vi "LumberjackConfigFromDTO.vi"(8 "error in (no error)":errorcluster, 11 "LumberjackConfigDTO":T9={"schemaVersion"="", "globalThreshold"="INFO", "defaultFileAppender"={"common"={"id"="", "threshold"="INFO", "filter"={"mode"="mirror", "levelMin"="INFO", "levelMax"="INFO", "tagPrefix"=""}, "queueBound"=0, "dropPolicy"="dropOldest", "useUTC"=FALSE}, "file"={"rootFolder"="", "maxFileSize"=0, "maxFileCount"=0, "baseName"="", "extension"="", "delimiter"="", "calendarFolderTree"=FALSE}}}) -> (0 "error out":errorcluster, 3 "LumberjackConfig":T1={"schemaVersion"="", "globalThreshold"=enum."INFO", "defaultFileAppender"={"common"={"id"="", "threshold"=enum."INFO", "filter"={"mode"=enum."Mirror", "levelMin"=enum."INFO", "levelMax"=enum."INFO", "tagPrefix"=""}, "queueBound"=0, "dropPolicy"=enum."DropOldest", "useUTC"=FALSE}, "file"={"rootFolder"=path "", "maxFileSize"=0, "maxFileCount"=0, "baseName"="", "extension"="", "delimiter"="", "calendarFolderTree"=FALSE}}})   [LabVIEW 2026, in "Lumberjack.lvlib"]
uses:
  Lumberjack.lvlib
  TypeDefs/Severity.ctl
  TypeDefs/FilterMode.ctl
  TypeDefs/Filter.ctl
  TypeDefs/DropPolicy.ctl
  TypeDefs/AppenderConfig.ctl
  TypeDefs/FileAppenderConfig.ctl
  TypeDefs/LumberjackConfig.ctl
  TypeDefs/FileConfig.ctl
  TypeDefs/ConfigDTO/FilterDTO.ctl
  TypeDefs/ConfigDTO/AppenderConfigDTO.ctl
  TypeDefs/ConfigDTO/FileAppenderConfigDTO.ctl
  TypeDefs/ConfigDTO/LumberjackConfigDTO.ctl
  TypeDefs/ConfigDTO/FileConfigDTO.ctl
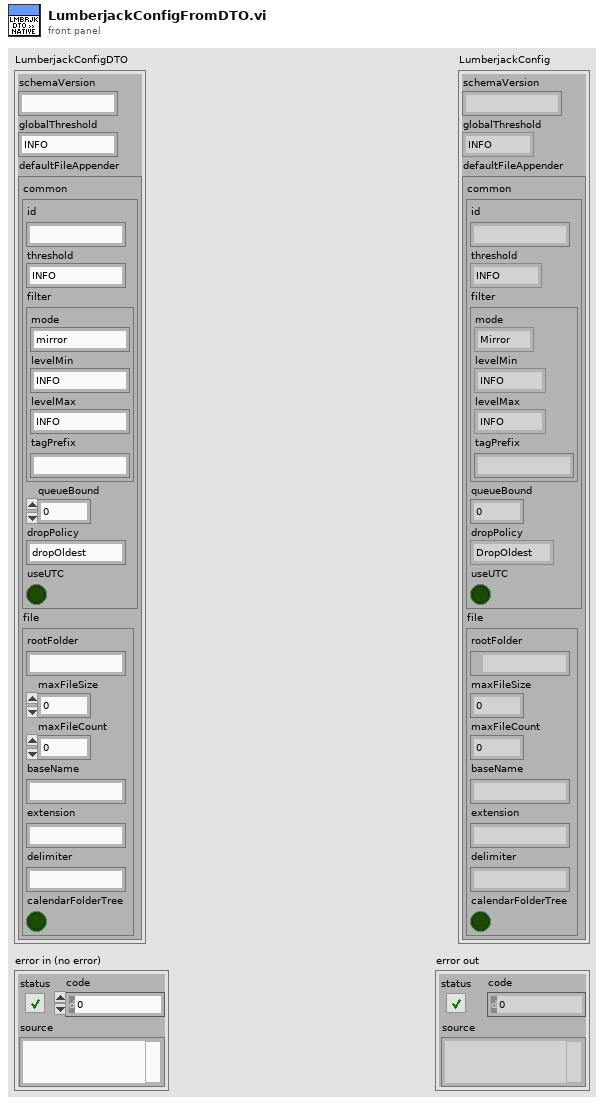
[diagram p1: front panel]
types:
  T1 = typedef "Lumberjack.lvlib/LumberjackConfig.ctl" = cluster{"schemaVersion":string, "globalThreshold":T2, "defaultFileAppender":T3}
  T2 = typedef "Lumberjack.lvlib/Severity.ctl" = enum16{"OFF", "FATAL", "ERROR", "WARN", "INFO", "DEBUG", "TRACE", "ALL"}
  T3 = typedef "Lumberjack.lvlib/FileAppenderConfig.ctl" = cluster{"common":T4, "file":T8}
  T4 = typedef "Lumberjack.lvlib/AppenderConfig.ctl" = cluster{"id":string, "threshold":T2, "filter":T5, "queueBound":i32, "dropPolicy":T7, "useUTC":bool}
  T5 = typedef "Lumberjack.lvlib/Filter.ctl" = cluster{"mode":T6, "levelMin":T2, "levelMax":T2, "tagPrefix":string}
  T6 = typedef "Lumberjack.lvlib/FilterMode.ctl" = enum16{"Mirror", "Routed"}
  T7 = typedef "Lumberjack.lvlib/DropPolicy.ctl" = enum16{"DropOldest", "DropNewest", "LevelAware"}
  T8 = typedef "Lumberjack.lvlib/FileConfig.ctl" = cluster{"rootFolder":path, "maxFileSize":i64, "maxFileCount":i32, "baseName":string, "extension":string, "delimiter":string, "calendarFolderTree":bool}
  T9 = typedef "Lumberjack.lvlib/LumberjackConfigDTO.ctl" = cluster{"schemaVersion":string, "globalThreshold":string, "defaultFileAppender":T10}
  T10 = typedef "Lumberjack.lvlib/FileAppenderConfigDTO.ctl" = cluster{"common":T11, "file":T13}
  T11 = typedef "Lumberjack.lvlib/AppenderConfigDTO.ctl" = cluster{"id":string, "threshold":string, "filter":T12, "queueBound":i32, "dropPolicy":string, "useUTC":bool}
  T12 = typedef "Lumberjack.lvlib/FilterDTO.ctl" = cluster{"mode":string, "levelMin":string, "levelMax":string, "tagPrefix":string}
  T13 = typedef "Lumberjack.lvlib/FileConfigDTO.ctl" = cluster{"rootFolder":string, "maxFileSize":i64, "maxFileCount":i32, "baseName":string, "extension":string, "delimiter":string, "calendarFolderTree":bool}
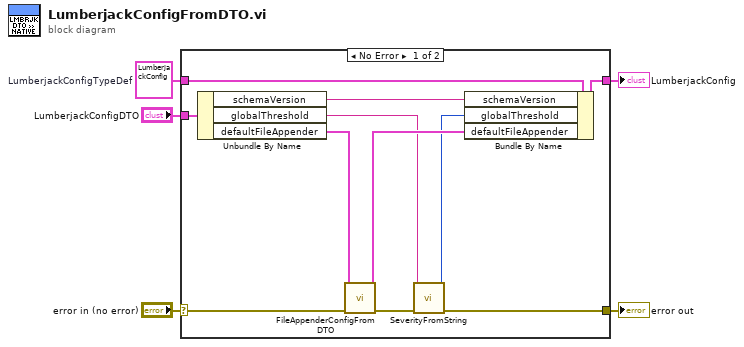
[diagram p0: block diagram]
diagram:
  w5 = T1 {"schemaVersion"="", "globalThreshold"=enum."INFO", "defaultFileAppender"={"common"={"id"="", "threshold"=enum."INFO", "filter"={"mode"=enum."Mirror", "levelMin"=enum."INFO", "levelMax"=enum."INFO", "tagPrefix"=""}, "queueBound"=0, "dropPolicy"=enum."DropOldest", "useUTC"=FALSE}, "file"={"rootFolder"=path "", "maxFileSize"=0, "maxFileCount"=0, "baseName"="", "extension"="", "delimiter"="", "calendarFolderTree"=FALSE}}}  # LumberjackConfigTypeDef
  n1 = case shown="No Error" "error in (no error)" {
    selector: "error in (no error)" -> [w16 w18]
    tunnel: [w10 w18] -> w4
    tunnel: "LumberjackConfigDTO" -> [w14 _]
    tunnel: [w15 w17] -> w2
    tunnel: w5 -> [w13 w17]
    frame No Error {
      n2 = Unbundle By Name(w14) -> ("schemaVersion"=w12:string, "globalThreshold"=w7:string, "defaultFileAppender"=w9:T10)
      n3 = call "FileAppenderConfigFromDTO.vi"("error in (no error)"=w16, "FileAppenderConfigDTO"=w9) -> ("error out"=w11:errorcluster, "FileAppenderConfig"=w8:T3)  [unwired: 8 in]
      n4 = call "SeverityFromString.vi"("error in (no error)"=w11, "SeverityString"=w7) -> ("error out"=w10:errorcluster, "Severity"=w6:T2)  [unwired: 8 in]
      n5 = Bundle By Name(cluster=w13, "schemaVersion"=w12, "globalThreshold"=w6, "defaultFileAppender"=w8) -> (w15:T1)
    }
    frame Error {
    }
  }
  "error out" <- w4
  "LumberjackConfig" <- w2
